vi "SetPrimaryButtonColors.vi"(8 "error in (no error)":errorcluster, 11 "Booleans":refnum<vi>[](array[refnum])) -> (0 "error out":errorcluster)   [LabVIEW 2024, in "Application.lvclass"]
uses:
  Application.lvclass
  Application.lvclass/Application.ctl
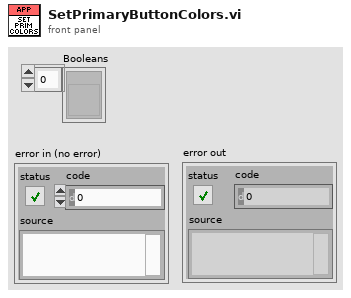
[diagram p1: front panel]
types:
  T1 = cluster{"ActiveBackground":u32, "ActiveBackground":u32}
  T2 = cluster{"PressedBackground":u32, "PressedBackground":u32}
  T3 = cluster{"DisabledBackground":u32, "DisabledBackground":u32}
  T4 = cluster{"DisabledBackground":u32, "DisabledBackground":u32}[]
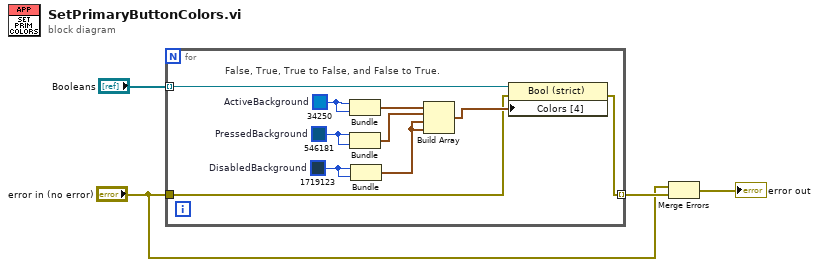
[diagram p0: block diagram]
diagram:
  n1 = for {
    tunnel: "Booleans" -> [w8] mode=indexing
    tunnel: "error in (no error)" -> [w6]
    tunnel: [w5] -> w3 mode=indexing
    w13 = u32 546181  # PressedBackground
    w12 = u32 1719123  # DisabledBackground
    w11 = u32 34250  # ActiveBackground
    # "False, True, True to False, and False to True."
    n2 = Bundle("ActiveBackground"=w11, "ActiveBackground"=w11) -> (w14:T1)  [unwired: 1 in]
    n3 = Bundle("PressedBackground"=w13, "PressedBackground"=w13) -> (w10:T2)  [unwired: 1 in]
    n4 = Bundle("DisabledBackground"=w12, "DisabledBackground"=w12) -> (w9:T3)  [unwired: 1 in]
    n5 = Build Array(w14, w10, w9, w9) -> (w7:T4)
    n6 = property class="Bool (strict)"(reference=w8, error in=w6, "Colors [4]"=w7) -> (error out=w5:errorcluster)  [unwired: 1 out]
  }
  n7 = Merge Errors("error in (no error)", w3) -> (→"error out":errorcluster)
